vi "Get Webdav.vi"(8 "error in (no error)":errorcluster, 10 "relative uri":string, 11 "Refnum in":T2) -> (0 "error out":errorcluster, 2 "file list":T1[](array[typedef]) caption="Dateiliste", 3 "session handle out":T2)   [LabVIEW 2019, in "SEECD System Explorer.lvlib"]
uses:
  SEECD System Explorer.lvlib
  <vilib>/WebDAVClient/Advanced/SessionHandle.ctl
  <vilib>/WebDAVClient/Advanced/FileInfo.ctl
  <vilib>/WebDAVClient/NI_WebDAV.lvlib
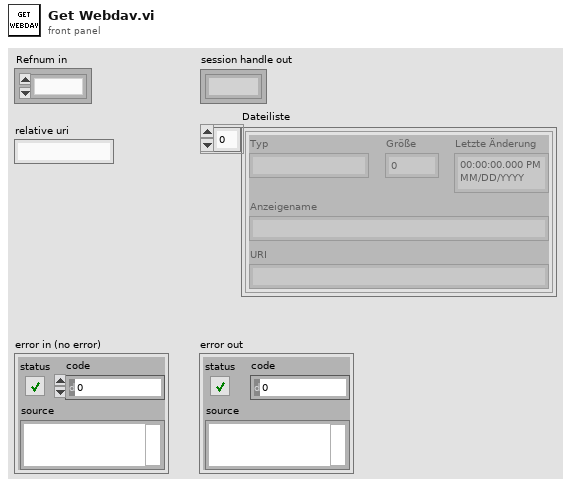
[diagram p1: front panel]
types:
  T1 = typedef "NI_WebDAV.lvlib/FileInfo.ctl" = cluster{"type":string, "size":u64, "last modification":timestamp, "display name":string, "uri":string}
  T2 = typedef "NI_WebDAV.lvlib/SessionHandle.ctl" = refnum<k1>
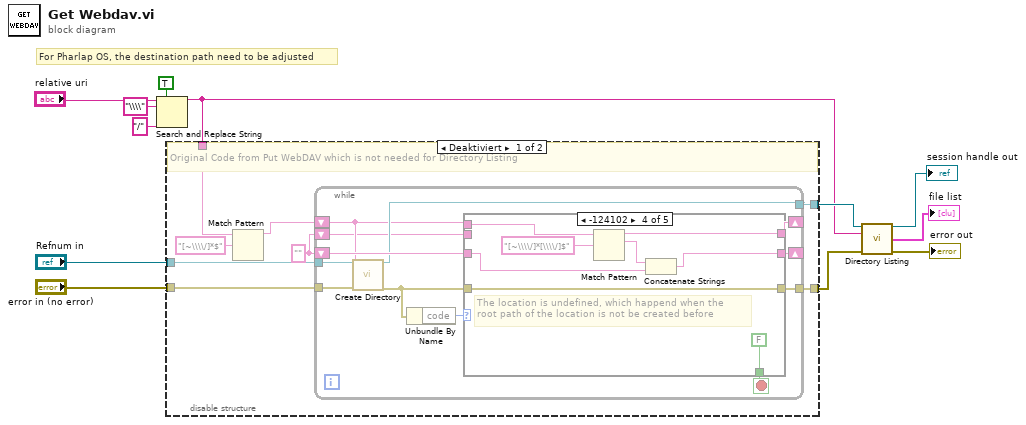
[diagram p0: block diagram]
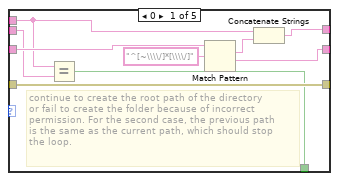
[diagram p2: hidden frame]
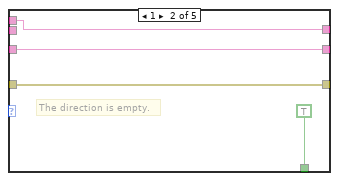
[diagram p3: hidden frame]
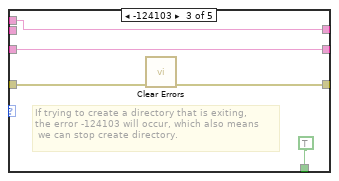
[diagram p4: hidden frame]
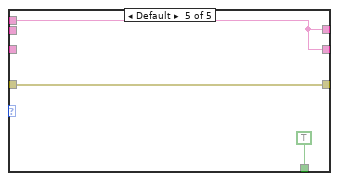
[diagram p5: hidden frame]
diagram:
  # "For Pharlap OS, the destination path need to be adjusted"
  n1 = Search and Replace String(replace all?=TRUE ("replace all? (F)"), input string="relative uri", search string="\\\\", replace string="/" ("replace string (\"\")")) -> (result string=w2:string)  [unwired: 4 in, 3 out]
  n2 = disable-structure shown="Deaktiviert" {
    disable-tunnel: [w20 w62] -> w11
    disable-tunnel: [w19 w63] -> w10
    disable-tunnel: "error in (no error)" -> [w18 w62]
    disable-tunnel: "Refnum in" -> [w17 w63]
    disable-tunnel: w2 -> [w15 _]
    frame Disabled {
      w13 = "" ("relative uri")
      # "Original Code from Put WebDAV which is not needed for Directory Listing"
      n3 = Match Pattern(string=w15, regular expression="[~\\\\/]*$") -> (before substring=w14:string)  [unwired: 1 in, 3 out]
      n4 = while {
        tunnel: w17 -> [w32]
        tunnel: w18 -> [w31]
        shift-right: [w30] -> _
        shift-left: w13 -> [w27]
        tunnel: [w26] -> w20
        shift-right: [w28] -> _
        shift-left: w13 -> [w21]
        tunnel: [w25] -> w19
        shift-left: w14 -> [w22]
        stop <- w29 stop-if-true
        n5 = call <vilib>:"Create Directory.vi"("session handle"=w32, "relative uri"=w22, "error in (no error)"=w31) -> ("session handle out"=w25:T2, "error out"=w23:errorcluster)  [unwired: 11 in]
        n6 = Unbundle By Name(w23) -> ("code"=w24:i32)
        n7 = case shown="-124102" w24 {
          tunnel: w22 -> [w35 w44 w49 w58 w60]
          tunnel: [w38 w43 w48 w55 w60] -> w30
          tunnel: [w33 TRUE TRUE FALSE TRUE] -> w29
          tunnel: [w39 w44 w49 w51 w60] -> w28
          tunnel: w27 -> [w36 w43 w48 w56 _]
          tunnel: w23 -> [w37 w42 w47 w53 w59]
          tunnel: [w37 w42 w46 w53 w59] -> w26
          tunnel: w21 -> [w34 _ _ _ _]
          frame 0 {
            # "continue to create the root path of the directory \nor fail to create the folder because of incorrect \npermission. For the second case, the previous path \nis the same as the current path, which should stop \nthe loop."
            n8 = Equal?(x=w35, y=w34) -> (x = y?=w33:bool)
            n9 = Match Pattern(string=w36, regular expression="^[~\\\\/]*[\\\\/]") -> (match substring=w40:string, after substring=w38:string)  [unwired: 1 in, 2 out]
            n10 = Concatenate Strings(w35, w40) -> (w39:string)
          }
          frame 1 {
            # "The direction is empty."
          }
          frame -124103 {
            # "If trying to create a directory that is exiting,\nthe error -124103 will occur, which also means\n we can stop create directory."
            n11 = call <vilib>:"Clear Errors.vi"("error in (no error)"=w47) -> ("error out"=w46:errorcluster)  [unwired: 5 in, 1 out]
          }
          frame -124102 {
            # "The location is undefined, which happend when the\nroot path of the location is not be created before"
            n12 = Match Pattern(string=w58, regular expression="[~\\\\/]*[\\\\/]$") -> (before substring=w51:string, match substring=w57:string)  [unwired: 1 in, 2 out]
            n13 = Concatenate Strings(w57, w56) -> (w55:string)
          }
          frame Default {
          }
        }
      }
    }
    frame Enabled {
    }
  }
  n14 = call <vilib>:"Directory Listing.vi"("session handle"=w10, "relative uri"=w2, "error in (no error)"=w11) -> ("session handle out"=→"session handle out":T2, "file list"=→"file list":T1[], "error out"=→"error out":errorcluster)  [unwired: 9 in, 1 out]
